vi "MoveTo.vi"(8 "error in (no error)":errorcluster, 9 "speed":string="400", 10 "positions":string[](array[string]), 11 "VISA Refnum in":refnum<visa-resource-name>) -> (0 "error out":errorcluster, 3 "VISA resource name out":refnum<visa-resource-name>)   [LabVIEW 2014, in "stepper3D.lvlib"]
uses:
  stepper3D.lvlib
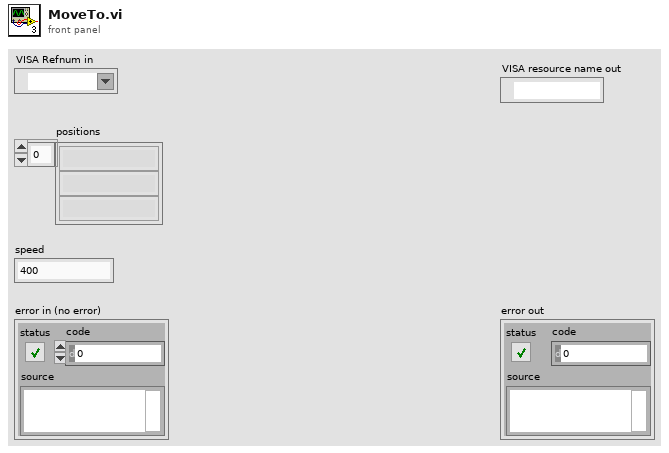
[diagram p1: front panel]
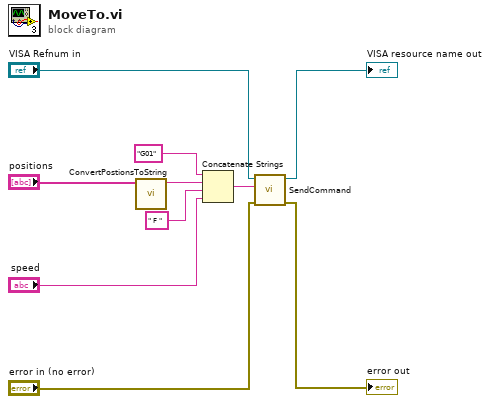
[diagram p0: block diagram]
diagram:
  n1 = call "ConvertPostionsToString.vi"("positions"="positions") -> ("output string"=w5:string)  [unwired: 10 in]
  n2 = Concatenate Strings("G01" ("command"), w5, " F " ("command"), "speed") -> (w4:string)
  n3 = call "SendCommand.vi"("error in (no error)"="error in (no error)", "command"=w4, "VISA Refnum in"="VISA Refnum in") -> ("error out"=→"error out":errorcluster, "VISA resource name out"=→"VISA resource name out":refnum<visa-resource-name>)  [unwired: 6 in, 1 out]
